vi "Motor cant move--error.vi"(10 "Direction":bool, 11 "Motor Speed":dbl) -> (0 "error out":errorcluster)   [LabVIEW 2024, in "Acquisition.lvlib"]
uses:
  Acquisition.lvlib
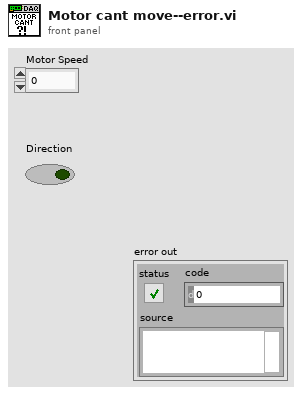
[diagram p1: front panel]
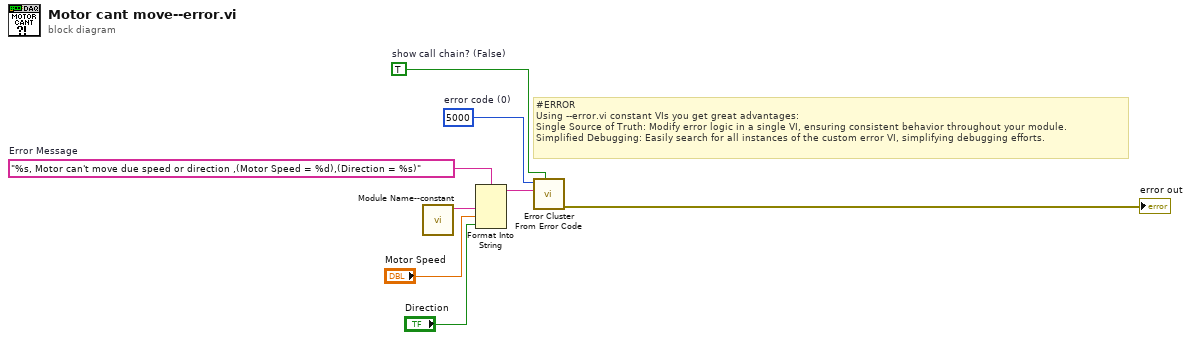
[diagram p0: block diagram]
diagram:
  w6 = 5000  # error code (0)
  w3 = "%s, Motor can't move due speed or direction ,(Motor Speed = %d),(Direction = %s)"  # Error Message
  w7 = TRUE  # show call chain? (False)
  # "#ERROR\nUsing --error.vi constant VIs you get great advantages:\nSingle Source of Truth: Modify error logic in a single VI, ensuring consistent behavior throughout your module.\nSimplified Debugging: Easily search for all instances of the custom error VI, simplifying debugging efforts."
  n1 = call "Module Name--constant.vi"() -> ("Module Name"=w5:string)  [unwired: 11 in]
  n2 = Format Into String(format string=w3, w5, "Motor Speed", "Direction") -> (resulting string=w4:string)  [unwired: 2 in, 1 out]
  n3 = call <vilib>:"Error Cluster From Error Code.vi"("show call chain? (False)"=w7, "error message (\"\")"=w4, "error code (0)"=w6) -> ("error out"=→"error out":errorcluster)  [unwired: 6 in]
